vi "GetTable.vi"(7 "LabVIEW Web Service Request":refnum<class "Web Request.lvclass">) -> (3 "xml string":string)   [LabVIEW 2016]
uses:
  <vilib>/wsapi/Web Request.lvclass
panel:
  # "Use the Web Service Request input terminal to call the VIs on the Web Services palette. Do not remove it from the connector pane unless you don't need access to the palette."
  # "Each additional control wired to the connector pane will be available as an input in the URL. To include an indicator in terminal-mode output (the default setting), it must also be wired to the connector pane."
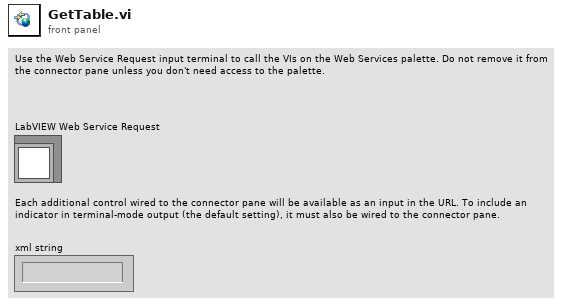
[diagram p1: front panel]
types:
  T1 = typedef "Array AE Data.ctl" = T2[]
  T2 = typedef "AE Data.ctl" = cluster{"Name":string, "Go?":bool, "Which batch?":enum16{"Anything", "First", "Second"}}
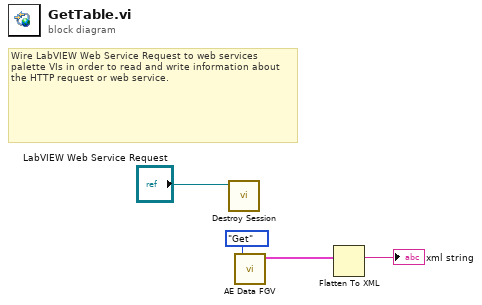
[diagram p0: block diagram]
diagram:
  # "Wire LabVIEW Web Service Request to web services palette VIs in order to read and write information about the HTTP request or web service."
  n1 = call <vilib>:"Destroy Session.vi"("LabVIEW Web Service Request"="LabVIEW Web Service Request") -> ()  [unwired: 13 in, 2 out]
  n2 = call "AE Data FGV.vi"("Command"=enum16{"Initialize", "Update", "Get"}."Get") -> ("Array of AEs"=w3:T1)  [unwired: 9 in, 1 out]
  n3 = Flatten To XML(anything=w3) -> (xml string=→"xml string":string)
